vi "Set Running Tests to Color.vi"(6 "Color":u32(colorbox)=16775978, 7 "FP Ref":refnum<vi>, 8 "Error In":errorcluster, 9 "Listbox Tests":string[](array[string]), 10 "Running Tests":string[](array[string]), 11 "Tests":refnum<vi>) -> (0 "Error Out":errorcluster)   [LabVIEW 2011]
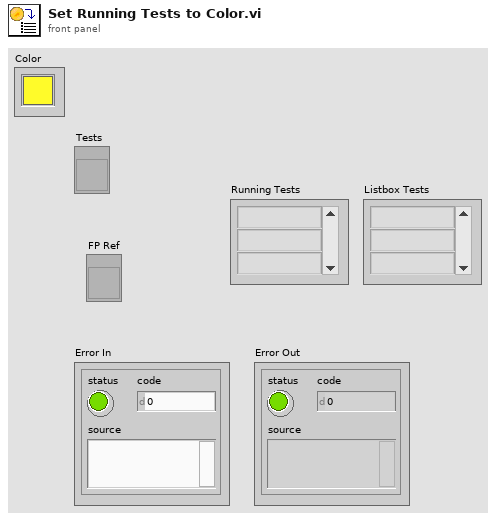
[diagram p1: front panel]
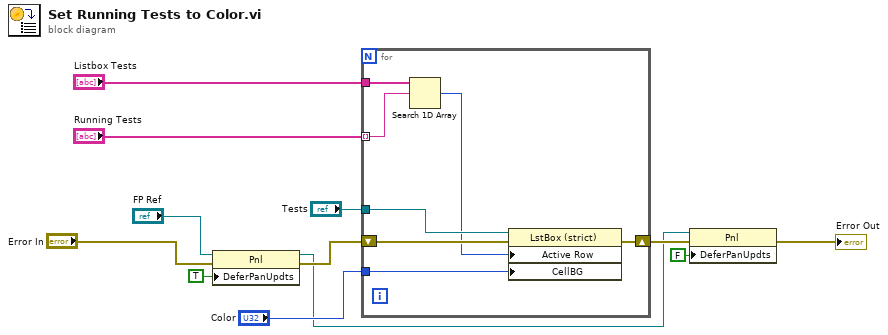
[diagram p0: block diagram]
diagram:
  n1 = property class="Pnl"(reference="FP Ref", error in="Error In", "DeferPanUpdts"=TRUE ("Defer Panel Updates")) -> (reference out=w5:refnum<vi>, error out=w9:errorcluster)
  n2 = for {
    tunnel: "Running Tests" -> [w18] mode=indexing
    tunnel: "Listbox Tests" -> [w19]
    tunnel: "Tests" -> [w16]
    tunnel: "Color" -> [w14]
    shift-right: [w13] -> w6
    shift-left: w9 -> [w17]
    n3 = Search 1D Array(1D array=w19, element=w18) -> (index of element=w15:i32)  [unwired: 1 in]
    n4 = property class="LstBox (strict)"(reference=w16, error in=w17, "Active Row"=w15, "CellBG"=w14) -> (error out=w13:errorcluster)  [unwired: 1 out]
  }
  n5 = property class="Pnl"(reference=w5, error in=w6, "DeferPanUpdts"=FALSE ("Defer Panel Updates")) -> (error out=→"Error Out":errorcluster)  [unwired: 1 out]
